vi "zad_12.vi"() -> ()   [LabVIEW 2024]
uses:
  Data_12.ctl
  <vilib>/regexp/Match Regular Expression.xnode
panel:
  out "error out":errorcluster
  in  "error in":errorcluster
  out "Limit exceeded?":bool
  out "To be moved":string
  in  "Sound intensity: MAX":dbl=100.0
  in  "Sound intensity: MIN":dbl
  in  "Stop":bool
  in  "Sound intensity [dB]":dbl(slide) scale=0.0..100.0
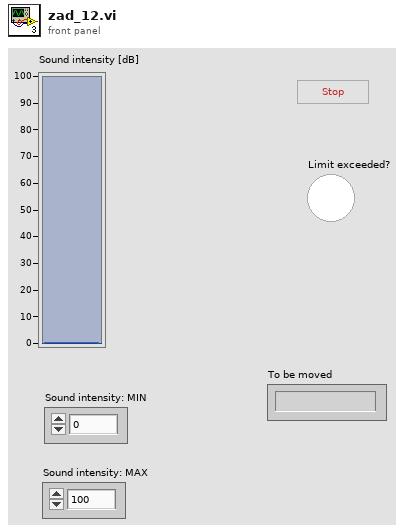
[diagram p1: front panel]
types:
  T1 = typedef "Data_12.ctl" = cluster{"Left":i32, "Top":i32, "Dragging":bool, "Letters":string}
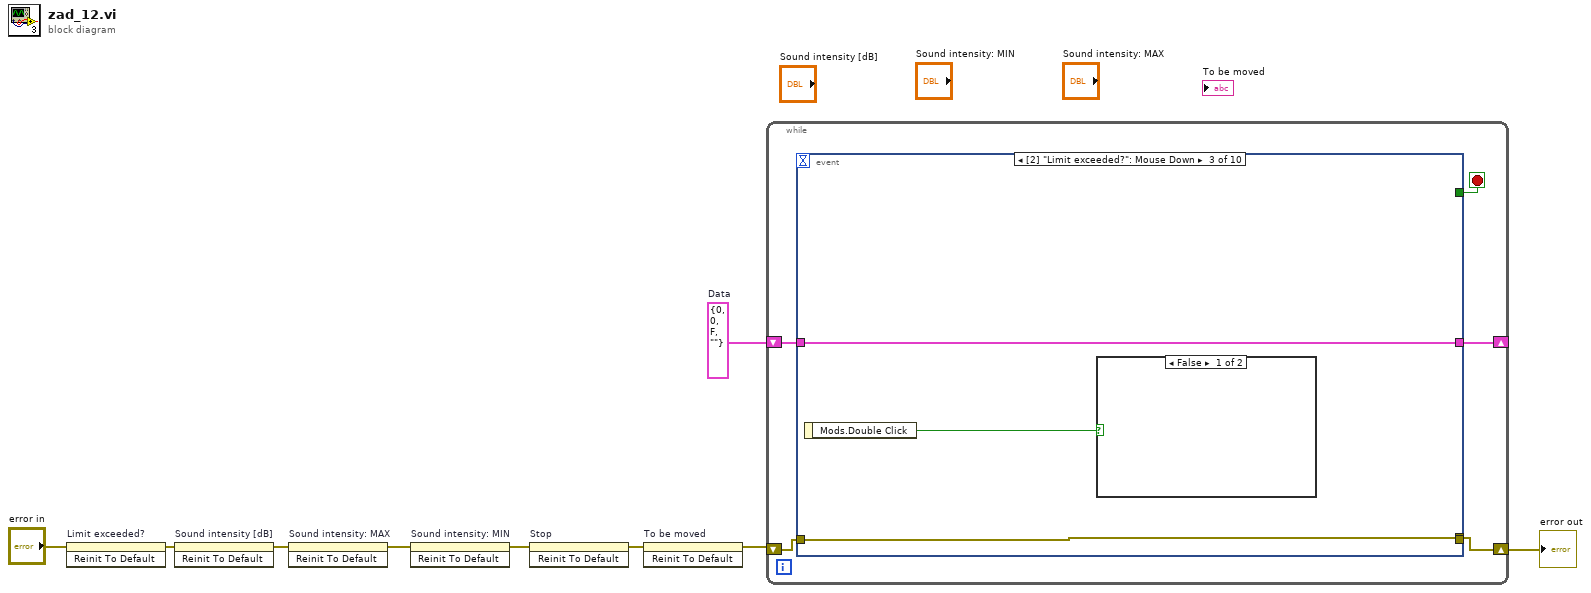
[diagram p0: block diagram]
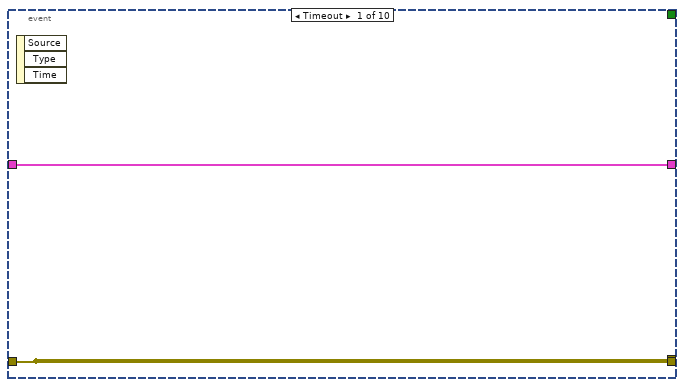
[diagram p2: hidden frame]
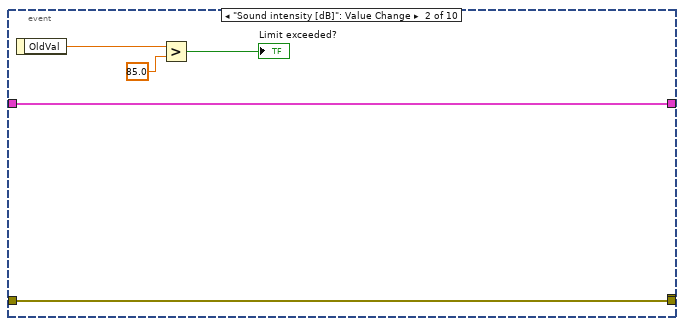
[diagram p3: hidden frame]
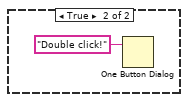
[diagram p4: hidden frame]
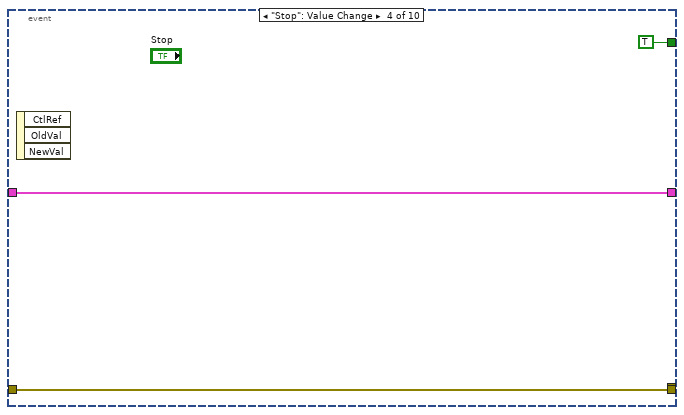
[diagram p5: hidden frame]
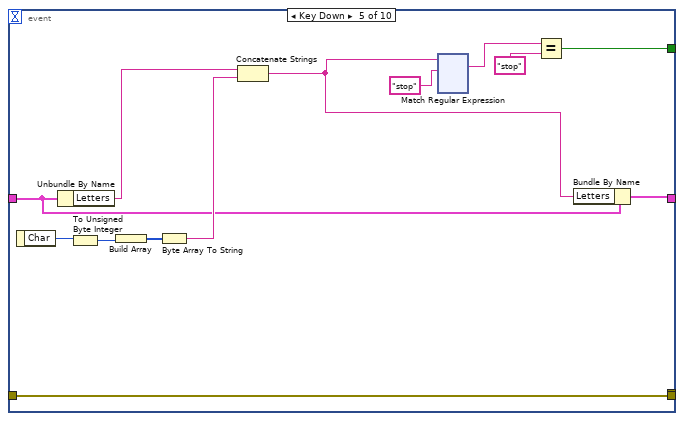
[diagram p6: hidden frame]
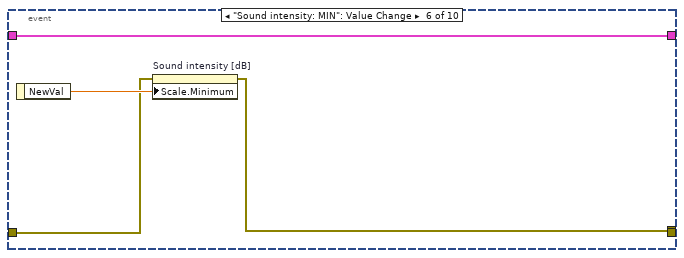
[diagram p7: hidden frame]
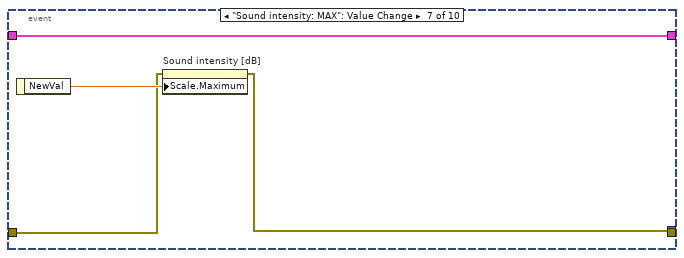
[diagram p8: hidden frame]
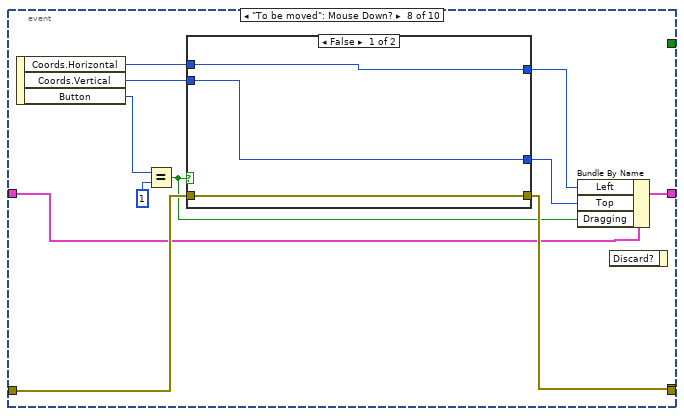
[diagram p9: hidden frame]
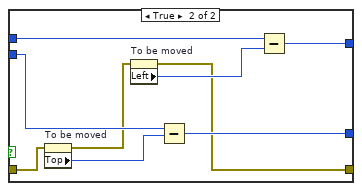
[diagram p10: hidden frame]
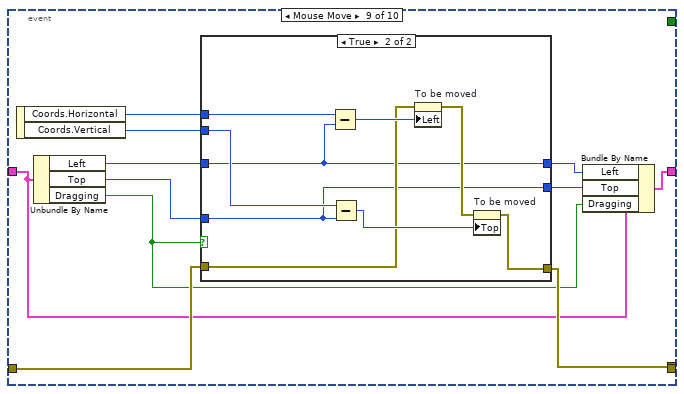
[diagram p11: hidden frame]
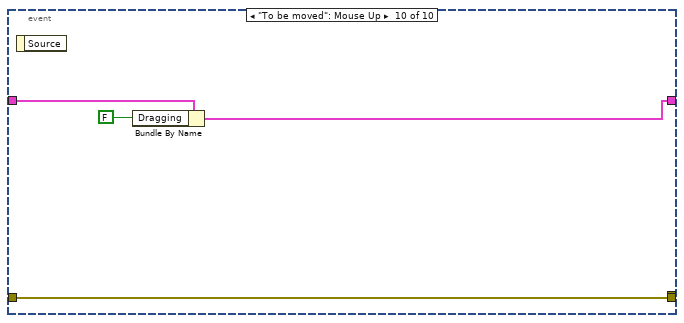
[diagram p13: hidden frame]
diagram:
  w1 = T1 {"Left"=0, "Top"=0, "Dragging"=FALSE, "Letters"=""}  # Data
  n1 = invoke on="Limit exceeded?" class="Bool (strict)" method="Reinit To Default"(error in="error in") -> (error out=w5:errorcluster)  [unwired: 2 in, 2 out]
  n2 = invoke on="Sound intensity [dB]" class="Slide (strict)" method="Reinit To Default"(error in=w5) -> (error out=w6:errorcluster)  [unwired: 2 in, 2 out]
  n3 = invoke on="Sound intensity: MAX" class="DigNum (strict)" method="Reinit To Default"(error in=w6) -> (error out=w7:errorcluster)  [unwired: 2 in, 2 out]
  n4 = invoke on="Sound intensity: MIN" class="DigNum (strict)" method="Reinit To Default"(error in=w7) -> (error out=w8:errorcluster)  [unwired: 2 in, 2 out]
  n5 = invoke on="Stop" class="Bool" method="Reinit To Default"(error in=w8) -> (error out=w9:errorcluster)  [unwired: 2 in, 2 out]
  n6 = invoke on="To be moved" class="Str" method="Reinit To Default"(error in=w9) -> (error out=w2:errorcluster)  [unwired: 2 in, 2 out]
  n7 = while {
    shift-right: [w12] -> w3
    shift-left: w2 -> [w13]
    shift-right: [w10] -> _
    shift-left: w1 -> [w11]
    stop <- w14 stop-if-true
    n8 = event shown="[2] \"Limit exceeded?\": Mouse Down" {
      selector: _ -> [_ _ _ _ _ _ _ _ _ _]
      dyn-events: _ -> [_ _ _ _ _ _ _ _ _ _]
      timeout: _ -> [_ _ _ _ _ _ _ _ _ _]
      tunnel: [_ _ _ TRUE w37 _ _ _ _ _] -> w14
      tunnel: w13 -> [w16 w18 w22 w27 w41 w161 w165 w173 w200 w216]
      tunnel: [w16 w18 w22 w27 w41 w160 w164 w172 w199 w216] -> w12
      tunnel: [w16 _ _ _ _ _ _ _ _ _] -> _
      tunnel: w11 -> [w15 w17 w23 w26 w31 w159 w163 w171 w194 w215]
      tunnel: [w15 w17 w23 w26 w29 w159 w163 w168 w191 w213] -> w10
      event Timeout {
        n9 = event-data() -> ()  [unwired: 1 in, 3 out]
      }
      event "Sound intensity [dB]": Value Change {
        n10 = event-data() -> ("OldVal"=w21:dbl)  [unwired: 1 in]
        n11 = Greater?(x=w21, y=85.0) -> (0:→"Limit exceeded?":bool)
      }
      event "Limit exceeded?": Mouse Down {
        n12 = event-data() -> ("Mods.Double Click"=w24:bool)  [unwired: 1 in]
        n13 = case shown="False" w24 {
          frame False {
          }
          frame True {
            n14 = One Button Dialog(message="Double click!") -> ()  [unwired: 1 in, 1 out]
          }
        }
      }
      event "Stop": Value Change {
        n15 = event-data() -> ()  [unwired: 1 in, 3 out]
      }
      event Key Down {
        n16 = event-data() -> ("Char"=w36:i16)  [unwired: 1 in]
        n17 = Unbundle By Name(w31) -> ("Letters"=w32:string)
        n18 = To Unsigned Byte Integer(number=w36) -> (unsigned 8bit integer=w35:u8)
        n19 = Build Array(w35) -> (w34:u8[])
        n20 = Byte Array To String(unsigned byte array=w34) -> (string=w33:string)
        n21 = Concatenate Strings(w32, w33) -> (w30:string)
        n22 = xnode "Match Regular Expression"("input string"=w30, "regular expression"="stop") -> ("whole match"=w39:string)  [unwired: 4 in, 4 out]
        n23 = Equal?(x=w39, y="stop") -> (x = y?=w37:bool)
        n24 = Bundle By Name(cluster=w31, "Letters"=w30) -> (w29:T1)
      }
      event "Sound intensity: MIN": Value Change {
        n25 = event-data() -> ("NewVal"=w162:dbl)  [unwired: 1 in]
        n26 = property on="Sound intensity [dB]" class="Slide (strict)"(error in=w161, "Scale.Minimum"=w162) -> (error out=w160:errorcluster)  [unwired: 1 in, 1 out]
      }
      event "Sound intensity: MAX": Value Change {
        n27 = event-data() -> ("NewVal"=w166:dbl)  [unwired: 1 in]
        n28 = property on="Sound intensity [dB]" class="Slide (strict)"(error in=w165, "Scale.Maximum"=w166) -> (error out=w164:errorcluster)  [unwired: 1 in, 1 out]
      }
      event "To be moved": Mouse Down? {
        n29 = event-data() -> ("Coords.Horizontal"=w177:i32, "Coords.Vertical"=w176:i32, "Button"=w175:u16)  [unwired: 1 in]
        n30 = Equal?(x=w175, y=u16 1) -> (x = y?=w167:bool)
        n31 = case shown="False" w167 {
          tunnel: w177 -> [w179 w189]
          tunnel: w176 -> [w180 w188]
          tunnel: [w180 w187] -> w170
          tunnel: [w179 w186] -> w169
          tunnel: w173 -> [w178 w183]
          tunnel: [w178 w181] -> w172
          frame False {
          }
          frame True {
            n32 = property on="To be moved" class="Str"(error in=w183) -> (error out=w182:errorcluster, "Top"=w184:i32)  [unwired: 1 in, 1 out]
            n33 = property on="To be moved" class="Str"(error in=w182) -> (error out=w181:errorcluster, "Left"=w185:i32)  [unwired: 1 in, 1 out]
            n34 = Subtract(x=w188, y=w184) -> (x-y=w187:i32)
            n35 = Subtract(x=w189, y=w185) -> (x-y=w186:i32)
          }
        }
        n36 = Bundle By Name(cluster=w171, "Left"=w169, "Top"=w170, "Dragging"=w167) -> (w168:T1)
        n37 = event-data() -> ()  [unwired: 2 in, 1 out]
      }
      event Mouse Move {
        n38 = event-data() -> ("Coords.Horizontal"=w198:i32, "Coords.Vertical"=w197:i32)  [unwired: 1 in]
        n39 = Unbundle By Name(w194) -> ("Left"=w196:i32, "Top"=w195:i32, "Dragging"=w190:bool)
        n40 = case shown="True" w190 {
          tunnel: w200 -> [w203 w207]
          tunnel: [w203 w212] -> w199
          tunnel: w198 -> [_ w211]
          tunnel: w197 -> [_ w210]
          tunnel: w196 -> [w202 w205]
          tunnel: w195 -> [w201 w204]
          tunnel: [w202 w205] -> w193
          tunnel: [w201 w204] -> w192
          frame False {
          }
          frame True {
            n41 = Subtract(x=w211, y=w205) -> (x-y=w209:i32)
            n42 = Subtract(x=w210, y=w204) -> (x-y=w208:i32)
            n43 = property on="To be moved" class="Str"(error in=w207, "Left"=w209) -> (error out=w206:errorcluster)  [unwired: 1 in, 1 out]
            n44 = property on="To be moved" class="Str"(error in=w206, "Top"=w208) -> (error out=w212:errorcluster)  [unwired: 1 in, 1 out]
          }
        }
        n45 = Bundle By Name(cluster=w194, "Left"=w193, "Top"=w192, "Dragging"=w190) -> (w191:T1)
      }
      event "To be moved": Mouse Up {
        n46 = event-data() -> ()  [unwired: 1 in, 1 out]
        n47 = Bundle By Name(cluster=w215, "Dragging"=FALSE) -> (w213:T1)
      }
    }
  }
  "error out" <- w3
